vi "VI Refnum Lifetime Test.vi"(8 "error in (no error)":errorcluster, 11 "Async Actor Example in":refnum<class "Async Methods Actor Example.lvclass">) -> (0 "error out":errorcluster, 3 "Async Actor Example out":refnum<class "Async Methods Actor Example.lvclass">)   [LabVIEW 2023, in "Async Methods Actor Example.lvlib" / "Async Methods Actor Example.lvclass"]
uses:
  Async Methods Actor Example.lvclass
  Async Methods Actor Example.lvclass/Async Methods Actor Example.ctl
panel:
  in  "Stop":bool
  out "String":string
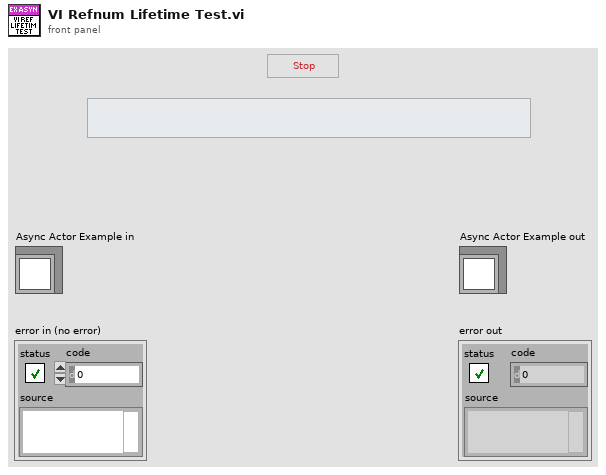
[diagram p1: front panel]
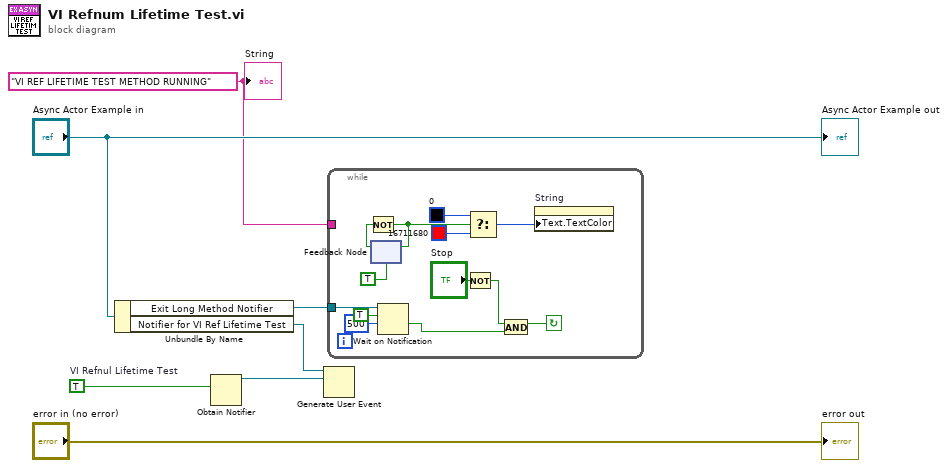
[diagram p0: block diagram]
diagram:
  w3 = TRUE  # VI Refnul Lifetime Test
  w4 = "VI REF LIFETIME TEST METHOD RUNNING" ("String")
  n1 = Unbundle By Name("Async Actor Example in") -> ("Exit Long Method Notifier"=w5:refnum<notifier>, "Notifier for VI Ref Lifetime Test"=w2:refnum<user-event>)
  n2 = Obtain Notifier(notification data type=w3) -> (notifier out=w1:refnum<notifier>)  [unwired: 3 in, 2 out]
  n3 = Generate User Event(user event=w2, event data cluster=w1) -> ()  [unwired: 2 in, 2 out]
  n4 = while {
    tunnel: w5 -> [w14]
    tunnel: w4 -> [_]
    stop <- w12 continue-if-true
    n5 = feedback #1(TRUE) -> (w19:bool)
    n6 = Not(x=w19) -> (.not. x?=w18:bool)
    n7 = feedback-in #1(w18) -> ()
    n8 = Wait on Notification(notifier=w14, ignore previous (F)=TRUE, timeout in ms (-1)=500) -> (timed out?=w11:bool)  [unwired: 1 in, 3 out]
    n9 = Not(x="Stop") -> (.not. x?=w9:bool)
    n10 = Select(t=u32 0 ("Text.Text Colors:Text Color"), s=w18, f=u32 16711680 ("Text.Text Colors:Text Color")) -> (s? t:f=w15:u32)
    n11 = And(x=w9, y=w11) -> (x .and. y?=w12:bool)
    n12 = property on="String" class="Str"("Text.TextColor"=w15) -> ()  [unwired: 2 in, 2 out]
  }
  "error out" <- "error in (no error)"
  "Async Actor Example out" <- "Async Actor Example in"
  "String" <- w4
